vi "Test_API_DelayedShutdown_PostShutdownEventsCaptured.vi"(8 "error in (no error)":errorcluster, 11 "TestCase in":refnum<class "TestLocalLogInstance.lvclass">) -> (0 "error out":errorcluster, 3 "TestCase out":refnum<class "TestLocalLogInstance.lvclass">)   [LabVIEW 2019, in "TestLocalLogInstance.lvclass"]
uses:
  TestLocalLogInstance.lvclass
  Source/Composed Log/Types/Log Level.ctl
  Source/Composed Log/LoggerReference/LoggerReference.lvclass/LoggerReference.ctl
  Source/LVQueue Sink/LVQueue Sink.lvclass/LVQueue Sink.ctl
  e881e85d-d289-450a-a3bf-8e76de4143bc.vi
  Source/Composed Log/LoggerReference/Return Aggregate Queues.vi
  Source/Composed Log/LoggerReference/Add Aggregate Log.vi
  e881e85d-d289-450a-a3bf-8e76de4143bc.vi/56849bd9-e0f3-42e2-9e62-1194216846a3.vi
  Source/Composed Log/LoggerReference/Log.vi
  Source/Composed Log/LoggerReference/Get Valid Event Time.vi
  Source/Composed Log/LoggerReference/Send Add Sink.vi
  Source/Composed Log/LoggerReference/Remove Stale Logs.vi
  Source/LVQueue Sink/LVQueue Sink.lvclass
  C:/CS/Log/Source/Composed Log/Log Sink/Log Sink.lvclass
  Source/Composed Log/Application Logger/Launch Worker Loop.vi
  Source/Composed Log/LoggerReference/Initialize Logger Instance.vi
  Source/Composed Log/LoggerReference/LoggerReference.lvclass
  Source/Composed Log/IErrorFormat/IErrorFormat.lvclass
  Source/Composed Log/Log Sink/Log Sink.lvclass
  <vilib>/addons/_JKI Toolkits/VI Tester/TestCase.llb/TestCase.lvclass
  Source/Composed Log/Composed Log.lvlib
  C:/Program Files (x86)/National Instruments/LabVIEW 2019/vi.lib/addons/_JKI Toolkits/VI Tester/TestCase.llb/TestCase.lvclass
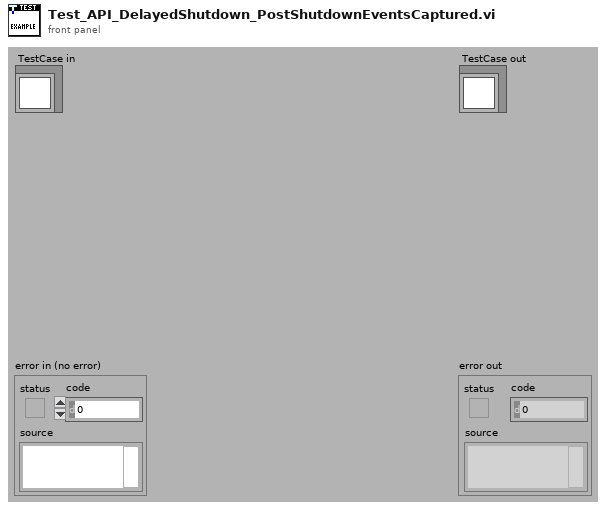
[diagram p1: front panel]
types:
  T1 = typedef "Composed Log.lvlib/Log Level.ctl" = enum16{"Debug", "Info", "Warning", "Error", "Critical"}
  T2 = typedef "Composed Log.lvlib/Log Packet.ctl" = cluster{"Data To Log":string, "Source":string, "Event Level":T1, "Event Time":timestamp}
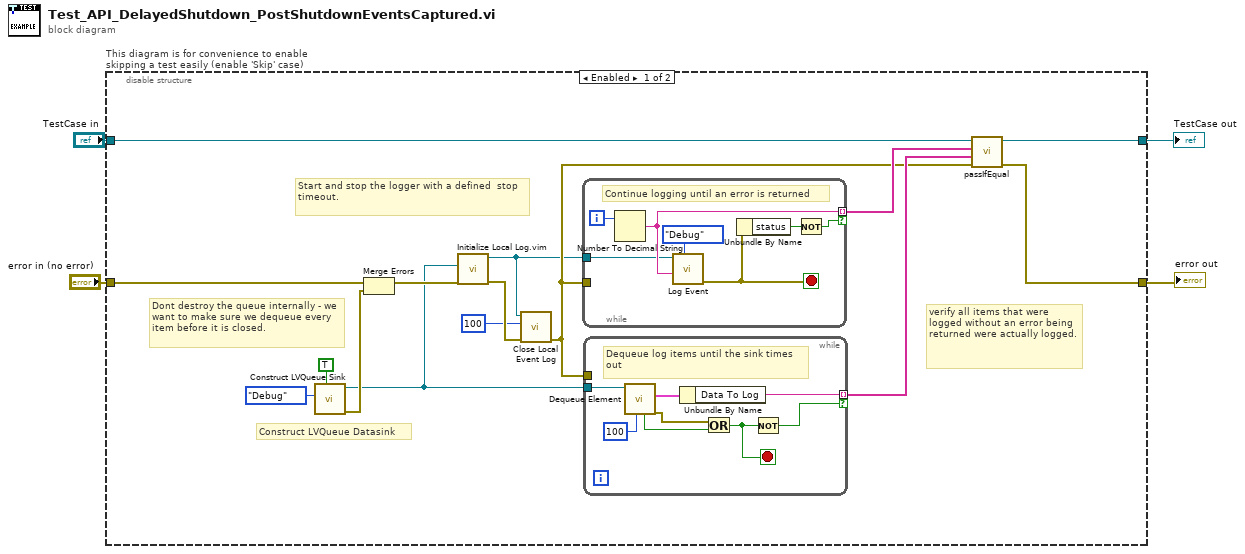
[diagram p0: block diagram]
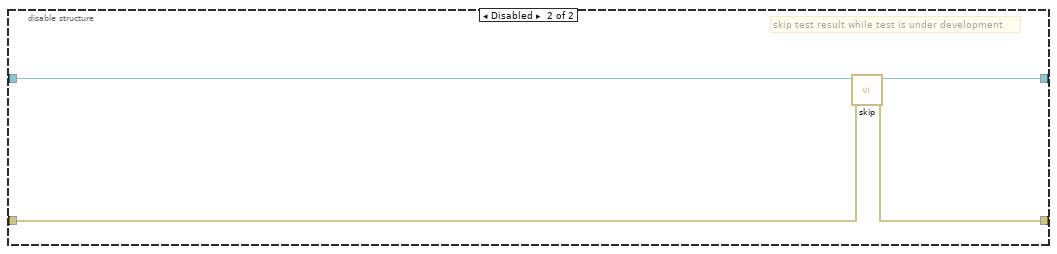
[diagram p2: hidden frame]
diagram:
  n1 = disable-structure "This diagram is for convenience to enable skipping a test easily (enable 'Skip' case)" shown="Enabled" {
    disable-tunnel: "TestCase in" -> [w17 w38]
    disable-tunnel: [w18 w36] -> w1
    disable-tunnel: [w16 w37] -> w3
    disable-tunnel: "error in (no error)" -> [w19 w35]
    frame Enabled {
      # "Dont destroy the queue internally - we want to make sure we dequeue every item before it is closed."
      # "verify all items that were logged without an error being returned were actually logged."
      # "Construct LVQueue Datasink"
      # "Start and stop the logger with a defined  stop timeout."
      n2 = call "Construct LVQueue Sink.vi"("User Shutdown? (F)"=TRUE, "LogLevel"=Log_Level."Debug") -> ("error out"=w14:errorcluster, "LVQueue Sink out"=w9:refnum<class "LVQueue Sink.lvclass">)  [unwired: 8 in]
      n3 = Merge Errors(w19, w14) -> (w10:errorcluster)
      n4 = call "Initialize Local Log.vim"("error in (no error)"=w10, "Startup Sink(s)"=w9) -> ("error out"=w8:errorcluster, "Log Instance Reference"=w5:refnum<class "LoggerReference.lvclass">)  [unwired: 7 in, 1 out]
      n5 = call "Close Local Event Log.vi"("error in (no error)"=w8, "Deferred Close Time (0 ms)"=u32 100 ("Deferred Close Time (ms)"), "Log Instance"=w5) -> ("error out"=w7:errorcluster)  [unwired: 8 in]
      n6 = while {
        tunnel: w7 -> [_]
        tunnel: [w29] -> w13 mode=indexing if=w30
        tunnel: w5 -> [w28]
        i -> [w33]
        stop <- w32 stop-if-true
        # "Continue logging until an error is returned"
        n7 = Number To Decimal String(number=w33) -> (decimal integer string=w29:string)  [unwired: 1 in]
        n8 = call "Log Event.vi"("Event Level"=Log_Level."Debug", "Data To Log"=w29, "Log Instance"=w28) -> ("error out"=w32:errorcluster)  [unwired: 7 in, 1 out]
        n9 = Unbundle By Name(w32) -> ("status"=w31:bool)
        n10 = Not(x=w31) -> (.not. x?=w30:bool)
      }
      n11 = while {
        tunnel: w9 -> [w27]
        tunnel: [w24] -> w11 mode=indexing if=w21
        tunnel: w7 -> [_]
        stop <- w20 stop-if-true
        # "Dequeue log items until the sink times out"
        n12 = call "Dequeue Element.vi"("timeout in ms (-1)"=100, "LVQueue Sink in"=w27) -> ("error out"=w22:errorcluster, "Log Packet"=w25:T2, "Timed Out?"=w23:bool)  [unwired: 6 in, 1 out]
        n13 = Unbundle By Name(w25) -> ("Data To Log"=w24:string)
        n14 = Or(x=w22, y=w23) -> (x .or. y?=w20:bool)
        n15 = Not(x=w20) -> (.not. x?=w21:bool)
      }
      n16 = call-dynamic "passIfEqual.vi"("error in (no error)"=w7, "y"=w11, "x"=w13, "TestCase in"=w17) -> ("error out"=w16:errorcluster, "TestCase out"=w18:refnum<class "TestLocalLogInstance.lvclass">)  [unwired: 6 in]
    }
    frame Disabled {
      # "skip test result while test is under development"
      n17 = call <vilib>:"skip.vi"("error in (no error)"=w35, "TestCase in"=w38) -> ("error out"=w37:errorcluster, "TestCase out"=w36:refnum<class "TestLocalLogInstance.lvclass">)  [unwired: 8 in]
    }
  }
  "error out" <- w3
  "TestCase out" <- w1
